vi "Restore Configuration.vi"(8 "error in (no error)":errorcluster, 10 "File path":path, 11 "Monitor-Pulse in":refnum<class "LabActor.lvclass">) -> (0 "error out":errorcluster, 1 "Section out":string, 2 "File path out":path, 3 "Monitor-Pulse out":refnum<class "LabActor.lvclass">)   [LabVIEW 2018, in "LabActor.lvclass"]
uses:
  LabActor.lvclass
  C:/github/LabActor/Controllers/Application Controller/Application Controller.lvclass
  Controllers/Application Controller/Application Controller.lvclass/Application Controller.ctl
  LabActor.lvclass/LabActor.ctl
  Controllers/Application Controller/Read Postproc ref.vi
  <vilib>/Utility/error.llb/Error Cluster From Error Code.vi
  NHMFL_Core/Libraries/Queued Listbox/Queued Listbox.xctl
  <vilib>/ErrorRing/Error Ring.xnode
  Controllers/Application Controller/Application Controller.lvclass
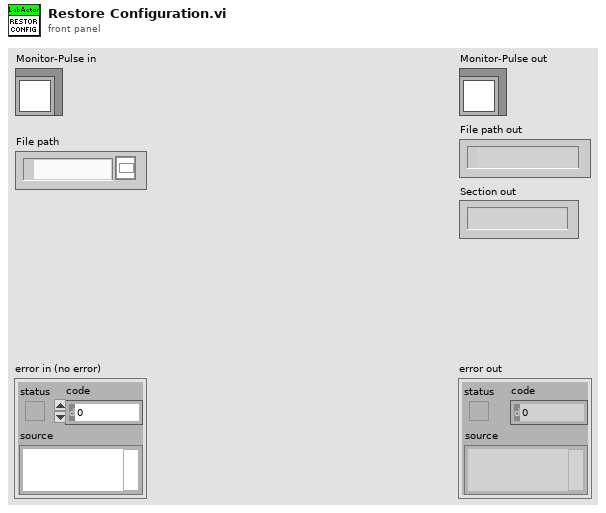
[diagram p1: front panel]
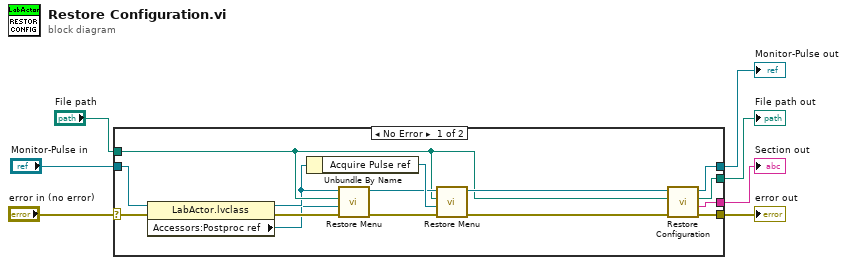
[diagram p0: block diagram]
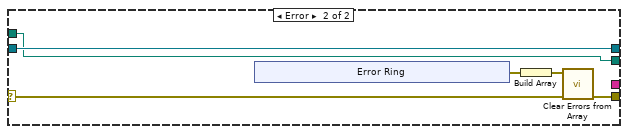
[diagram p2: hidden frame]
diagram:
  n1 = case shown="No Error" "error in (no error)" {
    selector: "error in (no error)" -> [w12 w24]
    tunnel: [w22 _] -> w7
    tunnel: [w21 w28] -> w6
    tunnel: "Monitor-Pulse in" -> [w10 w28]
    tunnel: [w20 w23] -> w4
    tunnel: [w19 w27] -> w3
    tunnel: "File path" -> [w13 w27]
    frame No Error {
      n2 = property class="LabActor.lvclass"(reference=w10, error in=w12) -> (reference out=w9:refnum<class "LabActor.lvclass">, error out=w11:errorcluster, "Accessors:Postproc ref"=w8:refnum<vi>)
      n3 = Unbundle By Name(w9) -> ("Acquire Pulse ref"=w16:refnum<vi>)
      n4 = call-dynamic "Restore Menu.vi"("error in (no error)"=w11, "Menu ref"=w8, "File path"=w13, "Monitor-Pulse in"=w9) -> ("error out"=w14:errorcluster, "Monitor-Pulse out"=w15:refnum<class "LabActor.lvclass">)  [unwired: 4 in, 2 out]
      n5 = call-dynamic "Restore Menu.vi"("error in (no error)"=w14, "Menu ref"=w16, "File path"=w13, "Monitor-Pulse in"=w15) -> ("error out"=w17:errorcluster, "Monitor-Pulse out"=w18:refnum<class "LabActor.lvclass">)  [unwired: 4 in, 2 out]
      n6 = call-parent "Restore Configuration.vi"("error in (no error)"=w17, "File path"=w13, "Measure Object in"=w18) -> ("error out"=w20:errorcluster, "Section out"=w22:string, "File path out"=w19:path, "Measure Object out"=w21:refnum<class "LabActor.lvclass">)  [unwired: 5 in]
    }
    frame Error {
      n7 = xnode "Error Ring"() -> ("error out"=w26:errorcluster)
      n8 = Build Array(w26) -> (w25:errorcluster[])
      n9 = call "Clear Errors from Array.vi"("Error In"=w24, "Errors to clear"=w25) -> ("Error Out"=w23:errorcluster)  [unwired: 8 in, 1 out]
    }
  }
  "error out" <- w4
  "Monitor-Pulse out" <- w6
  "File path out" <- w3
  "Section out" <- w7
